vi "Close.vi"(8 "error in":errorcluster, 11 "VISA resource name":refnum<visa-resource-name>) -> (0 "error out":errorcluster)   [LabVIEW 2020, in "HandsOnPi2040.lvlib"]
doc: "Performs an instrument error query before terminating the software connection to the instrument."
uses:
  HandsOnPi2040.lvlib
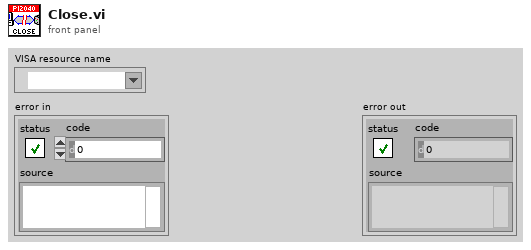
[diagram p1: front panel]
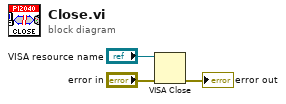
[diagram p0: block diagram]
diagram:
  n1 = VISA Close(VISA resource name="VISA resource name", error in (no error)="error in") -> (error out=→"error out":errorcluster)
